vi "DFD Inverse Chebyshev Design.vi"(4 "stopband atten [dB]":dbl=60.0 format="%.2f", 6 "fs [Hz]":dbl=1.0 format="%.2f", 7 "filter type":T1(ring), 8 "error in (no error)":errorcluster, 9 "low cutoff freq [Hz]":dbl=0.12, 10 "high cutoff freq [Hz]":dbl=0.45, 11 "order":i32=2) -> (0 "error out":errorcluster, 3 "filter out":T2={"mSRate_Fs"=1.0, "mSRate_Version"="2.0", "mSRate_Comments"="", "mSRate_OrgCoef"={"type"=enum."Undefined", "gain"=1.0, "coef a (k)"=[], "coef b (v)"=[]}, "mSRate_CurCoef"={"type"=enum."Undefined", "gain"=1.0, "coef a (k)"=[], "coef b (v)"=[]}, "mSRate_Quantized?"=FALSE, "mSRate_QCoef"={"type"=enum."Undefined", "gain"=1.0, "coef a (k)"=[], "coef b (v)"=[]}, "mSRate_QSettings"=[], "mSRate_Order"=0, "mSRate_Scaling"={"mSRate_ScaleByPowerOf2?"=FALSE, "mSRate_ScaleType"=enum."No Norm"}} {"mSRate_QSettings"."source" items=["Coef a/k"=0, "Coef b/v"=7, "Input"=1, "Output"=2, "Multiplicand"=3, "Product"=4, "Sum"=5, "Delay"=6, "Gain"=8]})   [LabVIEW 2017, in "NI_DigFilterLicensed.lvlib"]
doc: "Creates a digital Inverse Chebyshev infinite impulse response (IIR) filter."
uses:
  <vilib>/addons/Digital Filter Design/NI_DigFilterLicensed.lvlib
  <vilib>/addons/Digital Filter Design/_Objects.llb/DFD Filter Obj.ctl
  <vilib>/addons/Digital Filter Design/_Objects.llb/DFD Filter Coef.ctl
  <vilib>/addons/Digital Filter Design/_Objects.llb/DFD Filter Structure Type Selector.ctl
  <vilib>/addons/Digital Filter Design/_Objects.llb/dfd_Internal Quantization Settings.ctl
  <vilib>/addons/Digital Filter Design/_Objects.llb/dfd_Internal Quantization Srcs.ctl
  <vilib>/addons/Digital Filter Design/_Objects.llb/DFD Coef Norm Type.ctl
  <vilib>/addons/Digital Filter Design/NI_DigFilter_Design.lvlib
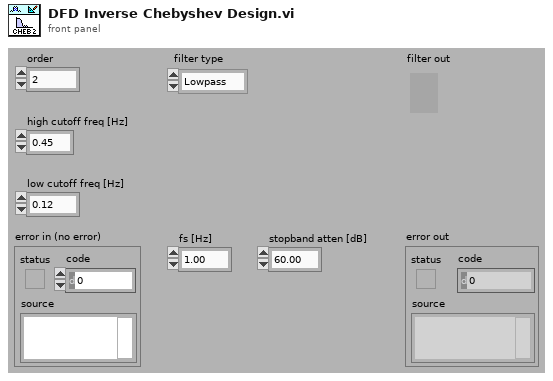
[diagram p1: front panel]
types:
  T1 = enum16{"Lowpass", "Highpass", "Bandpass", "Bandstop"}
  T2 = typedef "NI_DigFilterLicensed.lvlib/DFD Filter Obj.ctl" = cluster{"mSRate_Fs":dbl, "mSRate_Version":string, "mSRate_Comments":string, "mSRate_OrgCoef":T3, "mSRate_CurCoef":T3, "mSRate_Quantized?":bool, "mSRate_QCoef":T3, "mSRate_QSettings":T5[], "mSRate_Order":i32, "mSRate_Scaling":cluster{"mSRate_ScaleByPowerOf2?":bool, "mSRate_ScaleType":T7}}
  T3 = typedef "NI_DigFilterLicensed.lvlib/DFD Filter Coef.ctl" = cluster{"type":T4, "gain":dbl, "coef a (k)":dbl[], "coef b (v)":dbl[]}
  T4 = typedef "NI_DigFilterLicensed.lvlib/DFD Filter Structure Type Selector.ctl" = enum16{"Undefined", "FIR Direct Form", "FIR Direct Form Transposed", "FIR Symmetric", "FIR Antisymmetric", "IIR Direct Form I", "IIR Direct Form I Transposed", "IIR Direct Form II", "IIR Direct Form II Transposed", "IIR Cascaded Second Order Sections Form I", "IIR Cascaded Second Order Sections Form I Transposed", "IIR Cascaded Second Order Sections Form II", "IIR Cascaded Second Order Sections Form II Transposed", "Lattice Allpass (basic sections)", "Lattice Allpass (one multiplier sections)", "Lattice Allpass (normalized sections)", "Lattice AR (basic sections)", "Lattice AR (one multiplier sections)", "Lattice AR (normalized sections)", "Lattice MA (minimum phase)", "Lattice MA (maximum phase)", "Lattice ARMA (basic sections)", "Lattice ARMA (one multiplier sections)", "Lattice ARMA (normalized sections)"}
  T5 = typedef "NI_DigFilterLicensed.lvlib/dfd_Internal Quantization Settings.ctl" = cluster{"source":T6, "wl":i16, "iwl":i16, "overflow mode":enum16{"Saturation", "Wrap"}, "rounding mode":enum16{"Nearest", "Truncation"}, "signed?":bool}
  T6 = typedef "NI_DigFilterLicensed.lvlib/dfd_Internal Quantization Srcs.ctl" = u16
  T7 = typedef "NI_DigFilterLicensed.lvlib/DFD Coef Norm Type.ctl" = enum16{"No Norm", "Time Domain 1-Norm", "Time Domain 2-Norm", "Time Domain Inf-Norm"}
  T8 = enum16{"Butterworth", "Chebyshev", "Inv Chebyshev", "Elliptic", "Bessel"}
  T9 = cluster{"stopband atten [dB]":dbl, "stopband atten [dB]":dbl}
  T10 = typedef "NI_DigFilterLicensed.lvlib/DFD Pole-Zero.ctl" = cluster{"value":cdb, "z attr":cluster{"real":bool, "lp":bool, "uc":bool}, "order":i32}
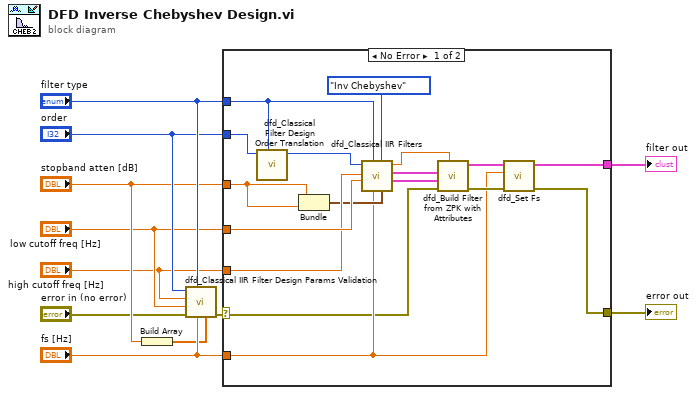
[diagram p0: block diagram]
diagram:
  n1 = Build Array("stopband atten [dB]") -> (w2:dbl[])
  n2 = call <vilib>:"dfd_Classical IIR Filter Design Params Validation.vi"("params"=w2, "fs [Hz]"="fs [Hz]", "filter type"="filter type", "error in (no error)"="error in (no error)", "low cutoff freq: fl"="low cutoff freq [Hz]", "high cutoff freq: fh"="high cutoff freq [Hz]", "order"="order") -> ("error out"=w1:errorcluster)  [unwired: 4 out]
  n3 = case shown="No Error" w1 {
    selector: w1 -> [w12 w29]
    tunnel: [w16 _] -> w11
    tunnel: [w15 w29] -> w10
    tunnel: "filter type" -> [w28 _]
    tunnel: "order" -> [w27 _]
    tunnel: "stopband atten [dB]" -> [w26 _]
    tunnel: "fs [Hz]" -> [w14 _]
    tunnel: "low cutoff freq [Hz]" -> [w25 _]
    tunnel: "high cutoff freq [Hz]" -> [w24 _]
    frame No Error {
      n4 = call <vilib>:"dfd_Classical Filter Design Order Translation.vi"("filter type"=w28, "input order"=w27) -> ("order for design"=w21:i32)  [unwired: 9 out]
      n5 = Bundle("stopband atten [dB]"=w26, "stopband atten [dB]"=w26) -> (w17:T9)  [unwired: 1 out]
      n6 = call <vilib>:"dfd_Classical IIR Filters.vi"("ripples [dB]"=w17, "filter design"=T8."Inv Chebyshev", "fs [Hz]"=w14, "filter type"=w28, "low cutoff freq: fl"=w25, "high cutoff freq: fh"=w24, "order"=w21) -> ("poles"=w13:T10[], "zeros"=w23:T10[], "gain"=w22:dbl)  [unwired: 2 in]
      n7 = call <vilib>:"dfd_Build Filter from ZPK with Attributes.vi"("gain"=w22, "error in (no error)"=w12, "poles"=w13, "zeros"=w23) -> ("error out"=w20:errorcluster, "filter out"=w19:T2)  [unwired: 6 out]
      n8 = call <vilib>:"dfd_Set Fs.vi"("error in (no error)"=w20, "fs [Hz]"=w14, "filter in"=w19) -> ("error out"=w15:errorcluster, "filter out"=w16:T2)  [unwired: 7 out]
    }
    frame Error {
    }
  }
  "filter out" <- w11
  "error out" <- w10
